vi "KelvinoxMonitor.vi"() -> ()   [LabVIEW 2019]
uses:
  Utility/Monitor Communication/Kelvinox/Kelvinox_Status_DD.ctl
  Global/Global Variables/Data_Display_global.vi
  Instrument_Setup.vi
panel:
  out "Kelvinox-Cluster":T1 {"Sorb Heater" format="%#.0f"; "Still Heater" format="%#.0f"; "MC Heater" format="%#.0f"; "T-Setpoint" format="%.3g"; "Sample" format="%_6g"; "4K" format="%_3g"; "MC" format="%_6g"; "Cold\nPlate" format="%_3g"; "1K Pot" format="%_3g"; "Still" format="%_3g"; "P5" format="%_3f"; "P4" format="%_3f"; "P3" format="%_3f"; "P2" format="%_3f"; "P1" format="%_3g"; "Dump" scale=0.0..1000.0}
  # "Hz"
  # "Temperatures in K"
  # "Resistances in Ohm"
  # "Pressures in mbar"
  # "Powers in µW"
  # "DU"
  # "He\nTrap"
  # "LN2\nTrap"
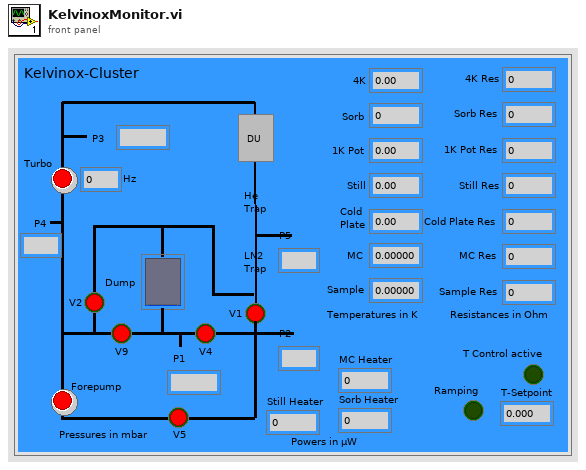
[diagram p1: front panel]
types:
  T1 = typedef "Kelvinox_Status_DD.ctl" = cluster{"V1":bool, "V2":bool, "Dump":u16, "V4":bool, "V5":bool, "V9":bool, "P1":dbl, "P2":dbl, "P3":dbl, "P4":dbl, "P5":dbl, "Turbo":bool, "Forepump":bool, "speed":dbl, "Sorb":dbl, "1K Pot":dbl, "Still":dbl, "Cold\nPlate":dbl, "MC":dbl, "4K":dbl, "Sample":dbl, "T-Setpoint":dbl, "MC Heater":dbl, "Still Heater":dbl, "Sorb Heater":dbl, "T Control active":bool, "Sorb Res":dbl, "1K Pot Res":dbl, "Still Res":dbl, "Cold Plate Res":dbl, "MC Res":dbl, "4K Res":dbl, "Sample Res":dbl, "Ramping":bool}
  T2 = cluster{"Mode":enum16{"Standard", "Buffered", "CRLF", "Immediate"}, "Bytes to Read":i32, "IP Address":string, "Remote Port":u16, "Timeout":i32, "connection ID":refnum<k5>}
  T3 = typedef "Kelvinox_Status.ctl" = cluster{"V1":bool, "V2":bool, "Dump":u16, "V4":bool, "V5":bool, "V9":bool, "P1":dbl, "P2":dbl, "P3":dbl, "P4":dbl, "P5":dbl, "Turbo":bool, "Forepump":bool, "speed":dbl, "Sorb":dbl, "1K Pot":dbl, "Still":dbl, "Cold\nPlate":dbl, "MC":dbl, "4K":dbl, "Sample":dbl, "T-Setpoint":dbl, "MC Heater":dbl, "Still Heater":dbl, "Sorb Heater":dbl, "T Control active":bool, "Sorb Res":dbl, "1K Pot Res":dbl, "Still Res":dbl, "Cold Plate Res":dbl, "MC Res":dbl, "4K Res":dbl, "Sample Res":dbl, "Ramping":bool}
  T4 = cluster{"Mode":enum16{"Standard", "Buffered", "CRLF", "Immediate"}, "Bytes to Read":i32, "IP Address":string, "Remote Port":i32, "Timeout":i32, "connection ID":refnum<k5>}
  T5 = typedef "Kelvinox_Control.ctl" = cluster{"T-Setpoint-Manual":dbl, "Rate (K/min)":dbl, "Change T Control Status":bool, "Emergency Stop":bool, "Set Setpoint":bool}
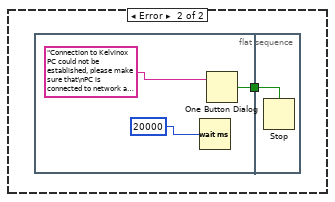
[diagram p2: hidden frame]
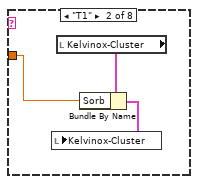
[diagram p4: hidden frame]
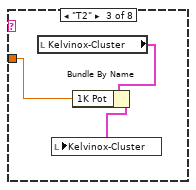
[diagram p5: hidden frame]
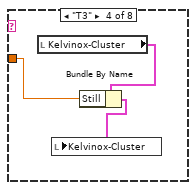
[diagram p6: hidden frame]
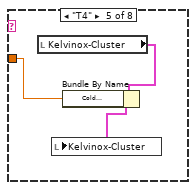
[diagram p7: hidden frame]
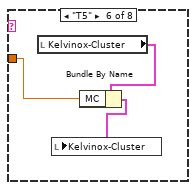
[diagram p8: hidden frame]
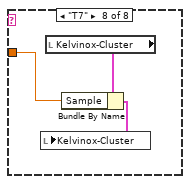
[diagram p9: hidden frame]
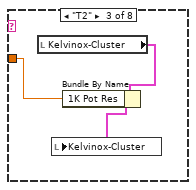
[diagram p11: hidden frame]
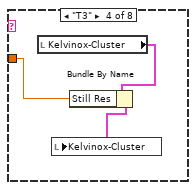
[diagram p12: hidden frame]
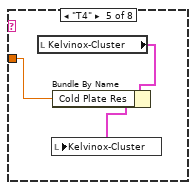
[diagram p13: hidden frame]
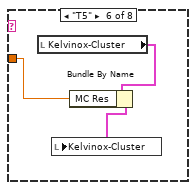
[diagram p14: hidden frame]
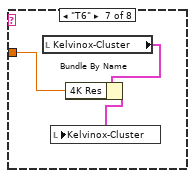
[diagram p15: hidden frame]
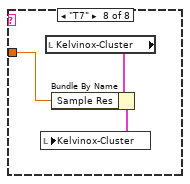
[diagram p16: hidden frame]
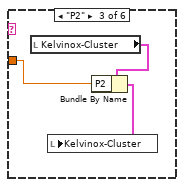
[diagram p18: hidden frame]
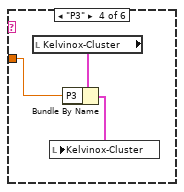
[diagram p19: hidden frame]
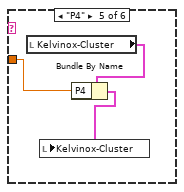
[diagram p20: hidden frame]
diagram:
  n1 = flat-sequence {
    tunnel: [w5] -> w3
    tunnel: [w4] -> w2
    tunnel: w3 -> [w14]
    tunnel: w2 -> [w13]
    tunnel: [w13] -> w1
    tunnel: w1 -> [w424]
    frame #0 {
      # "Establish TCP Connection"
      n2 = global read "Instrument_Setup.vi" "Connection Details Kelvinox"() -> (w6:T2)
      n3 = global read "Data_Display_global.vi" "Kelvinox-Cluster"() -> (→"Kelvinox-Cluster":T3)
      n4 = call "TRITON_RI_OPEN.vi"("Connection Details (in)"=w6) -> ("error out"=w5:errorcluster, "Connection Details (out)"=w4:T4)  [unwired: 2 in]
      n5 = case shown="No Error" w5 {
        frame No Error {
        }
        frame Error {
          n6 = flat-sequence {
            tunnel: [w9] -> w8
            tunnel: w8 -> [w12]
            frame #0 {
              n7 = Wait (ms)(milliseconds to wait=20000) -> ()  [unwired: 1 out]
              n8 = One Button Dialog(message="Connection to Kelvinox PC could not be established, please make sure that\nPC is connected to network and Triton control software is running.\n\nThe Kelvinox monitor will be restarted in 20 seconds if the status monitor is not stopped meanwhile.") -> (true=w9:bool)  [unwired: 1 in]
            }
            frame #1 {
              n9 = Stop(stop? (T)=w12) -> ()
            }
          }
        }
      }
    }
    frame #1 {
      n10 = while {
        tunnel: w14 -> [w40]
        tunnel: w13 -> [w41]
        stop <- w37 stop-if-true
        n11 = flat-sequence {
          tunnel: [w48] -> w36
          tunnel: [w50] -> w34
          tunnel: w40 -> [w49]
          tunnel: w41 -> [w50]
          tunnel: w36 -> [w89]
          tunnel: [w86] -> w35
          tunnel: w34 -> [w88]
          tunnel: [w88] -> w33
          tunnel: [w125] -> w47
          tunnel: [w124] -> w46
          tunnel: w35 -> [w126]
          tunnel: w33 -> [w124]
          tunnel: w47 -> [w161]
          tunnel: w46 -> [w158]
          tunnel: [w158] -> w45
          tunnel: [w157] -> w44
          tunnel: w45 -> [w195]
          tunnel: w44 -> [w199]
          tunnel: [w195] -> w43
          tunnel: [w193] -> w42
          tunnel: w43 -> [w206]
          tunnel: w42 -> [w210]
          tunnel: [w206] -> w32
          tunnel: [w205] -> w30
          tunnel: [w204] -> w28
          tunnel: w32 -> [w220]
          tunnel: [w220] -> w31
          tunnel: w30 -> [w216]
          tunnel: [w215] -> w29
          tunnel: w28 -> [w217]
          tunnel: w31 -> [w228]
          tunnel: [w228] -> w39
          tunnel: w29 -> [w230]
          tunnel: [w227] -> w38
          tunnel: w39 -> [w256]
          tunnel: [w256] -> w21
          tunnel: w38 -> [w257]
          tunnel: [w255] -> w19
          tunnel: [w254] -> w17
          tunnel: w21 -> [w266]
          tunnel: [w266] -> w20
          tunnel: w19 -> [w267]
          tunnel: [w268] -> w18
          tunnel: w17 -> [w269]
          tunnel: [w269] -> w16
          tunnel: [w264] -> w15
          tunnel: w20 -> [w282]
          tunnel: [w282] -> w25
          tunnel: w18 -> [w280]
          tunnel: [w281] -> w23
          tunnel: w16 -> [w283]
          tunnel: w15 -> [w276]
          tunnel: w25 -> [w292]
          tunnel: [w292] -> w24
          tunnel: w23 -> [w294]
          tunnel: [w293] -> w22
          tunnel: w24 -> [w388]
          tunnel: [w388] -> w27
          tunnel: w22 -> [w393]
          tunnel: [w395] -> w26
          tunnel: w27 -> [_]
          tunnel: w26 -> [w413]
          frame #0 {
            w51 = string[] ["T1", "T2", "T3", "T4", "T5", "T6", "T7"]
            # "Read Temperature Sensors"
            n12 = Array Size(array=w51) -> (size(s)=w52:i32)
            n13 = for {
              N: w52 -> [_]
              tunnel: w51 -> [w55] mode=indexing
              tunnel: w50 -> [w58]
              shift-right: [w56] -> w48
              shift-left: w49 -> [w57]
              n14 = Concatenate Strings("READ:DEV:", w55, ":TEMP:SIG:TEMP", "\r\n") -> (w64:string)
              n15 = call "TRITON_SEND_RECEIVE.vi"("error in (no error)"=w57, "Command String"=w64, "Communication Cluster"=w58) -> ("error out"=w60:errorcluster, "Response String"=w59:string)  [unwired: 1 in]
              n16 = call "TRITON_GET_VALUE.vi"("error in (no error)"=w60, "Response String"=w59) -> ("error out"=w56:errorcluster, "Value"=w54:dbl)  [unwired: 1 in, 1 out]
              n17 = case shown="\"T6\"" w55 {
                tunnel: w54 -> [_ w65 w68 w71 w74 w77 w82 w85]
                frame "empty", Default {
                }
                frame "T1" {
                  n18 = local read "Kelvinox-Cluster"() -> (w67:T1)
                  n19 = Bundle By Name(cluster=w67, "Sorb"=w65) -> (w66:T1)
                  n20 = local write "Kelvinox-Cluster"(w66) -> ()
                }
                frame "T2" {
                  n21 = local read "Kelvinox-Cluster"() -> (w70:T1)
                  n22 = Bundle By Name(cluster=w70, "1K Pot"=w68) -> (w69:T1)
                  n23 = local write "Kelvinox-Cluster"(w69) -> ()
                }
                frame "T3" {
                  n24 = local read "Kelvinox-Cluster"() -> (w73:T1)
                  n25 = Bundle By Name(cluster=w73, "Still"=w71) -> (w72:T1)
                  n26 = local write "Kelvinox-Cluster"(w72) -> ()
                }
                frame "T4" {
                  n27 = local read "Kelvinox-Cluster"() -> (w76:T1)
                  n28 = Bundle By Name(cluster=w76, "Cold\nPlate"=w74) -> (w75:T1)
                  n29 = local write "Kelvinox-Cluster"(w75) -> ()
                }
                frame "T5" {
                  n30 = local read "Kelvinox-Cluster"() -> (w79:T1)
                  n31 = Bundle By Name(cluster=w79, "MC"=w77) -> (w78:T1)
                  n32 = local write "Kelvinox-Cluster"(w78) -> ()
                }
                frame "T6" {
                  n33 = local read "Kelvinox-Cluster"() -> (w81:T1)
                  n34 = Bundle By Name(cluster=w81, "4K"=w82) -> (w80:T1)
                  n35 = local write "Kelvinox-Cluster"(w80) -> ()
                }
                frame "T7" {
                  n36 = local read "Kelvinox-Cluster"() -> (w84:T1)
                  n37 = Bundle By Name(cluster=w84, "Sample"=w85) -> (w83:T1)
                  n38 = local write "Kelvinox-Cluster"(w83) -> ()
                }
              }
              n39 = Wait (ms)(milliseconds to wait=10) -> ()  [unwired: 1 out]
            }
          }
          frame #1 {
            w87 = string[] ["T1", "T2", "T3", "T4", "T5", "T6", "T7"]
            # "Read Temperature Sensor Resistances"
            n40 = Array Size(array=w87) -> (size(s)=w90:i32)
            n41 = for {
              N: w90 -> [_]
              tunnel: w87 -> [w93] mode=indexing
              tunnel: w88 -> [w96]
              shift-right: [w94] -> w86
              shift-left: w89 -> [w95]
              n42 = Concatenate Strings("READ:DEV:", w93, ":TEMP:SIG:RES", "\r\n") -> (w102:string)
              n43 = call "TRITON_SEND_RECEIVE.vi"("error in (no error)"=w95, "Command String"=w102, "Communication Cluster"=w96) -> ("error out"=w98:errorcluster, "Response String"=w97:string)  [unwired: 1 in]
              n44 = call "TRITON_GET_VALUE.vi"("error in (no error)"=w98, "Response String"=w97) -> ("error out"=w94:errorcluster, "Value"=w92:dbl)  [unwired: 1 in, 1 out]
              n45 = case shown="\"T1\"" w93 {
                tunnel: w92 -> [_ w103 w106 w109 w112 w115 w120 w123]
                frame "empty", Default {
                }
                frame "T1" {
                  n46 = local read "Kelvinox-Cluster"() -> (w105:T1)
                  n47 = Bundle By Name(cluster=w105, "Sorb Res"=w103) -> (w104:T1)
                  n48 = local write "Kelvinox-Cluster"(w104) -> ()
                }
                frame "T2" {
                  n49 = local read "Kelvinox-Cluster"() -> (w108:T1)
                  n50 = Bundle By Name(cluster=w108, "1K Pot Res"=w106) -> (w107:T1)
                  n51 = local write "Kelvinox-Cluster"(w107) -> ()
                }
                frame "T3" {
                  n52 = local read "Kelvinox-Cluster"() -> (w111:T1)
                  n53 = Bundle By Name(cluster=w111, "Still Res"=w109) -> (w110:T1)
                  n54 = local write "Kelvinox-Cluster"(w110) -> ()
                }
                frame "T4" {
                  n55 = local read "Kelvinox-Cluster"() -> (w114:T1)
                  n56 = Bundle By Name(cluster=w114, "Cold Plate Res"=w112) -> (w113:T1)
                  n57 = local write "Kelvinox-Cluster"(w113) -> ()
                }
                frame "T5" {
                  n58 = local read "Kelvinox-Cluster"() -> (w117:T1)
                  n59 = Bundle By Name(cluster=w117, "MC Res"=w115) -> (w116:T1)
                  n60 = local write "Kelvinox-Cluster"(w116) -> ()
                }
                frame "T6" {
                  n61 = local read "Kelvinox-Cluster"() -> (w119:T1)
                  n62 = Bundle By Name(cluster=w119, "4K Res"=w120) -> (w118:T1)
                  n63 = local write "Kelvinox-Cluster"(w118) -> ()
                }
                frame "T7" {
                  n64 = local read "Kelvinox-Cluster"() -> (w122:T1)
                  n65 = Bundle By Name(cluster=w122, "Sample Res"=w123) -> (w121:T1)
                  n66 = local write "Kelvinox-Cluster"(w121) -> ()
                }
              }
              n67 = Wait (ms)(milliseconds to wait=10) -> ()  [unwired: 1 out]
            }
          }
          frame #2 {
            w128 = string[] ["P1", "P2", "P3", "P4", "P5"]
            # "Read Pressure Sensors"
            n68 = Array Size(array=w128) -> (size(s)=w127:i32)
            n69 = for {
              N: w127 -> [_]
              tunnel: w128 -> [w135] mode=indexing
              tunnel: w124 -> [w137]
              shift-right: [w132] -> w125
              shift-left: w126 -> [w136]
              n70 = Concatenate Strings("READ:DEV:", w135, ":PRES:SIG:PRES", "\r\n") -> (w140:string)
              n71 = call "TRITON_SEND_RECEIVE.vi"("error in (no error)"=w136, "Command String"=w140, "Communication Cluster"=w137) -> ("error out"=w133:errorcluster, "Response String"=w130:string)  [unwired: 1 in]
              n72 = call "TRITON_GET_VALUE.vi"("error in (no error)"=w133, "Response String"=w130) -> ("error out"=w132:errorcluster, "Value"=w131:dbl)  [unwired: 1 in, 1 out]
              n73 = case shown="\"P1\"" w135 {
                tunnel: w131 -> [_ w142 w145 w149 w151 w154]
                frame "empty", Default {
                }
                frame "P1" {
                  # "Nominal Dump\npressure:\n0.755 bar"
                  n74 = local read "Kelvinox-Cluster"() -> (w144:T1)
                  n75 = To Unsigned Word Integer(number=w142) -> (unsigned 16bit integer=w141:u16)
                  n76 = Bundle By Name(cluster=w144, "P1"=w142, "Dump"=w141) -> (w143:T1)
                  n77 = local write "Kelvinox-Cluster"(w143) -> ()
                }
                frame "P2" {
                  n78 = local read "Kelvinox-Cluster"() -> (w147:T1)
                  n79 = Bundle By Name(cluster=w147, "P2"=w145) -> (w146:T1)
                  n80 = local write "Kelvinox-Cluster"(w146) -> ()
                }
                frame "P3" {
                  n81 = local read "Kelvinox-Cluster"() -> (w150:T1)
                  n82 = Bundle By Name(cluster=w150, "P3"=w149) -> (w148:T1)
                  n83 = local write "Kelvinox-Cluster"(w148) -> ()
                }
                frame "P4" {
                  n84 = local read "Kelvinox-Cluster"() -> (w153:T1)
                  n85 = Bundle By Name(cluster=w153, "P4"=w151) -> (w152:T1)
                  n86 = local write "Kelvinox-Cluster"(w152) -> ()
                }
                frame "P5" {
                  n87 = local read "Kelvinox-Cluster"() -> (w156:T1)
                  n88 = Bundle By Name(cluster=w156, "P5"=w154) -> (w155:T1)
                  n89 = local write "Kelvinox-Cluster"(w155) -> ()
                }
              }
              n90 = Wait (ms)(milliseconds to wait=10) -> ()  [unwired: 1 out]
            }
          }
          frame #3 {
            w160 = string[] ["V1", "V2", "V4", "V5", "V9"]
            # "Read Valve States"
            n91 = Array Size(array=w160) -> (size(s)=w159:i32)
            n92 = for {
              N: w159 -> [_]
              shift-right: [w164] -> w157
              shift-left: w161 -> [w170]
              tunnel: w160 -> [w168] mode=indexing
              tunnel: w158 -> [w171]
              n93 = Concatenate Strings("READ:DEV:", w168, ":VALV:SIG:STATE", "\r\n") -> (w174:string)
              n94 = call "TRITON_SEND_RECEIVE.vi"("error in (no error)"=w170, "Command String"=w174, "Communication Cluster"=w171) -> ("error out"=w165:errorcluster, "Response String"=w166:string)  [unwired: 1 in]
              n95 = call "TRITON_GET_STATUS.vi"("error in (no error)"=w165, "Response String"=w166) -> ("error out"=w164:errorcluster, "Status"=w163:string)  [unwired: 2 in]
              n96 = call "Parse_Valve.vi"("Valve"=w163) -> ("Status"=w167:bool)
              n97 = case shown="\"V1\"" w168 {
                tunnel: w167 -> [w175 w178 w181 w184 w187 _]
                frame "V1" {
                  n98 = local read "Kelvinox-Cluster"() -> (w177:T1)
                  n99 = Bundle By Name(cluster=w177, "V1"=w175) -> (w176:T1)
                  n100 = local write "Kelvinox-Cluster"(w176) -> ()
                }
                frame "V2" {
                  n101 = local read "Kelvinox-Cluster"() -> (w180:T1)
                  n102 = Bundle By Name(cluster=w180, "V2"=w178) -> (w179:T1)
                  n103 = local write "Kelvinox-Cluster"(w179) -> ()
                }
                frame "V4" {
                  n104 = local read "Kelvinox-Cluster"() -> (w183:T1)
                  n105 = Bundle By Name(cluster=w183, "V4"=w181) -> (w182:T1)
                  n106 = local write "Kelvinox-Cluster"(w182) -> ()
                }
                frame "V5" {
                  n107 = local read "Kelvinox-Cluster"() -> (w186:T1)
                  n108 = Bundle By Name(cluster=w186, "V5"=w184) -> (w185:T1)
                  n109 = local write "Kelvinox-Cluster"(w185) -> ()
                }
                frame "V9" {
                  n110 = local read "Kelvinox-Cluster"() -> (w189:T1)
                  n111 = Bundle By Name(cluster=w189, "V9"=w187) -> (w188:T1)
                  n112 = local write "Kelvinox-Cluster"(w188) -> ()
                }
                frame "empty", Default {
                }
              }
              n113 = Wait (ms)(milliseconds to wait=10) -> ()  [unwired: 1 out]
            }
          }
          frame #4 {
            # "Read Forepump Status"
            n114 = Concatenate Strings("READ:DEV:FP:PUMP:SIG:STATE", "\r\n") -> (w202:string)
            n115 = call "TRITON_SEND_RECEIVE.vi"("error in (no error)"=w199, "Command String"=w202, "Communication Cluster"=w195) -> ("error out"=w194:errorcluster, "Response String"=w192:string)  [unwired: 1 in]
            n116 = call "TRITON_GET_STATUS.vi"("error in (no error)"=w194, "Response String"=w192) -> ("error out"=w193:errorcluster, "Status"=w191:string)  [unwired: 2 in]
            n117 = call "Parse_Valve.vi"("Valve"=w191) -> ("Status"=w197:bool)
            n118 = local read "Kelvinox-Cluster"() -> (w198:T1)
            n119 = Bundle By Name(cluster=w198, "Forepump"=w197) -> (w196:T1)
            n120 = local write "Kelvinox-Cluster"(w196) -> ()
            n121 = Wait (ms)(milliseconds to wait=10) -> ()  [unwired: 1 out]
          }
          frame #5 {
            # "Read Turbo Status"
            n122 = Concatenate Strings("READ:DEV:TURB1:PUMP:SIG:STATE", "\r\n") -> (w213:string)
            n123 = call "TRITON_SEND_RECEIVE.vi"("error in (no error)"=w210, "Command String"=w213, "Communication Cluster"=w206) -> ("error out"=w208:errorcluster, "Response String"=w209:string)  [unwired: 1 in]
            n124 = call "TRITON_GET_STATUS.vi"("error in (no error)"=w208, "Response String"=w209) -> ("error out"=w205:errorcluster, "Status"=w207:string)  [unwired: 2 in]
            n125 = call "Parse_Valve.vi"("Valve"=w207) -> ("Status"=w204:bool)
            n126 = Wait (ms)(milliseconds to wait=10) -> ()  [unwired: 1 out]
          }
          frame #6 {
            # "Read Turbo Speed"
            n127 = Concatenate Strings("READ:DEV:TURB1:PUMP:SIG:SPD", "\r\n") -> (w221:string)
            n128 = call "TRITON_SEND_RECEIVE.vi"("error in (no error)"=w216, "Command String"=w221, "Communication Cluster"=w220) -> ("error out"=w222:errorcluster, "Response String"=w223:string)  [unwired: 1 in]
            n129 = local read "Kelvinox-Cluster"() -> (w219:T1)
            n130 = call "TRITON_GET_VALUE.vi"("error in (no error)"=w222, "Response String"=w223) -> ("error out"=w215:errorcluster, "Value"=w224:dbl)  [unwired: 1 in, 1 out]
            n131 = Bundle By Name(cluster=w219, "Turbo"=w217, "speed"=w224) -> (w218:T1)
            n132 = local write "Kelvinox-Cluster"(w218) -> ()
            n133 = Wait (ms)(milliseconds to wait=10) -> ()  [unwired: 1 out]
          }
          frame #7 {
            w229 = string[] ["H1", "H2", "H3"]
            # "Read Heater Outputs"
            n134 = Array Size(array=w229) -> (size(s)=w231:i32)
            n135 = for {
              N: w231 -> [_]
              shift-right: [w237] -> w227
              shift-left: w230 -> [w239]
              tunnel: w229 -> [w234] mode=indexing
              tunnel: w228 -> [w238]
              n136 = Concatenate Strings("READ:DEV:", w234, ":HTR:SIG:POWR", "\r\n") -> (w243:string)
              n137 = call "TRITON_SEND_RECEIVE.vi"("error in (no error)"=w239, "Command String"=w243, "Communication Cluster"=w238) -> ("error out"=w236:errorcluster, "Response String"=w235:string)  [unwired: 1 in]
              n138 = call "TRITON_GET_VALUE.vi"("error in (no error)"=w236, "Response String"=w235) -> ("error out"=w237:errorcluster, "Value"=w233:dbl)  [unwired: 1 in, 1 out]
              n139 = case shown="\"H3\"" w234 {
                tunnel: w233 -> [w244 w247 w251 _]
                frame "H1" {
                  n140 = local read "Kelvinox-Cluster"() -> (w246:T1)
                  n141 = Bundle By Name(cluster=w246, "MC Heater"=w244) -> (w245:T1)
                  n142 = local write "Kelvinox-Cluster"(w245) -> ()
                }
                frame "H2" {
                  n143 = local read "Kelvinox-Cluster"() -> (w249:T1)
                  n144 = Bundle By Name(cluster=w249, "Still Heater"=w247) -> (w248:T1)
                  n145 = local write "Kelvinox-Cluster"(w248) -> ()
                }
                frame "H3" {
                  n146 = local read "Kelvinox-Cluster"() -> (w252:T1)
                  n147 = Bundle By Name(cluster=w252, "Sorb Heater"=w251) -> (w250:T1)
                  n148 = local write "Kelvinox-Cluster"(w250) -> ()
                }
                frame "empty", Default {
                }
              }
              n149 = Wait (ms)(milliseconds to wait=10) -> ()  [unwired: 1 out]
            }
          }
          frame #8 {
            # "Read Temperature Control"
            n150 = Concatenate Strings("READ:DEV:T5:TEMP:LOOP:MODE", "\r\n") -> (w263:string)
            n151 = call "TRITON_SEND_RECEIVE.vi"("error in (no error)"=w257, "Command String"=w263, "Communication Cluster"=w256) -> ("error out"=w259:errorcluster, "Response String"=w260:string)  [unwired: 1 in]
            n152 = call "TRITON_GET_STATUS.vi"("error in (no error)"=w259, "Response String"=w260) -> ("error out"=w255:errorcluster, "Status"=w258:string)  [unwired: 2 in]
            n153 = call "Parse_Valve.vi"("Valve"=w258) -> ("Status"=w254:bool)
            n154 = Wait (ms)(milliseconds to wait=10) -> ()  [unwired: 1 out]
          }
          frame #9 {
            # "Read Ramping Status"
            n155 = Concatenate Strings("READ:DEV:T5:TEMP:LOOP:RAMP:RAMPING", "\r\n") -> (w275:string)
            n156 = call "TRITON_SEND_RECEIVE.vi"("error in (no error)"=w267, "Command String"=w275, "Communication Cluster"=w266) -> ("error out"=w271:errorcluster, "Response String"=w272:string)  [unwired: 1 in]
            n157 = call "TRITON_GET_STATUS.vi"("error in (no error)"=w271, "Response String"=w272) -> ("error out"=w268:errorcluster, "Status"=w265:string)  [unwired: 2 in]
            n158 = Wait (ms)(milliseconds to wait=10) -> ()  [unwired: 1 out]
            n159 = call "Parse_Valve.vi"("Valve"=w265) -> ("Status"=w264:bool)
          }
          frame #10 {
            # "Read Temperature Control Setpoint"
            n160 = Concatenate Strings("READ:DEV:T5:TEMP:LOOP:TSET", "\r\n") -> (w289:string)
            n161 = call "TRITON_SEND_RECEIVE.vi"("error in (no error)"=w280, "Command String"=w289, "Communication Cluster"=w282) -> ("error out"=w284:errorcluster, "Response String"=w285:string)  [unwired: 1 in]
            n162 = local read "Kelvinox-Cluster"() -> (w279:T1)
            n163 = call "TRITON_GET_VALUE.vi"("error in (no error)"=w284, "Response String"=w285) -> ("error out"=w281:errorcluster, "Value"=w286:dbl)  [unwired: 1 in, 1 out]
            n164 = Bundle By Name(cluster=w279, "T Control active"=w283, "Ramping"=w276, "T-Setpoint"=w286) -> (w278:T1)
            n165 = local write "Kelvinox-Cluster"(w278) -> ()
            n166 = Wait (ms)(milliseconds to wait=10) -> ()  [unwired: 1 out]
          }
          frame #11 {
            # "ToDo: Implement Thermometer excitation and range"
            # "Change Heater Range if Loop mode is enabled"
            n167 = local read "Kelvinox-Cluster"() -> (w295:T1)
            n168 = Unbundle By Name(w295) -> ("T-Setpoint"=w290:dbl, "T Control active"=w291:bool)
            n169 = case shown="True" w291 {
              tunnel: w294 -> [w296 w311]
              tunnel: [w296 w310] -> w293
              tunnel: w292 -> [_ w309]
              tunnel: w290 -> [_ w306]
              frame False {
              }
              frame True {
                n170 = stacked-sequence {
                  seq-local: [w314 _ _ _] -> [_ w324 _ _]
                  seq-local: [_ w323 _ _] -> [_ _ w331 _]
                  seq-local: [_ _ w330 _] -> [_ _ _ w339]
                  tunnel: w311 -> [w319 _ _ _]
                  tunnel: w309 -> [w315 w322 w329 w337]
                  tunnel: [_ w320 _ _] -> w303
                  tunnel: [w312 _ _ _] -> w304
                  tunnel: [_ _ w328 _] -> w302
                  tunnel: [_ _ _ w336] -> w307
                  tunnel: [_ _ _ w338] -> w301
                  frame #0 {
                    n171 = Concatenate Strings("READ:DEV:T5:TEMP:LOOP:RANGE", "\r\n") -> (w316:string)
                    n172 = call "TRITON_SEND_RECEIVE.vi"("error in (no error)"=w319, "Command String"=w316, "Communication Cluster"=w315) -> ("error out"=w314:errorcluster, "Response String"=w313:string)  [unwired: 1 in]
                    n173 = call "Kelvinox_Parse_Heater_Excitation_to_Number.vi"("Excitation String"=w313) -> ("Excitation Level"=w312:dbl)
                  }
                  frame #1 {
                    n174 = Concatenate Strings("READ:DEV:T5:TEMP:LOOP:P", "\r\n") -> (w325:string)
                    n175 = call "TRITON_SEND_RECEIVE.vi"("error in (no error)"=w324, "Command String"=w325, "Communication Cluster"=w322) -> ("error out"=w323:errorcluster, "Response String"=w321:string)  [unwired: 1 in]
                    n176 = call "Kelvinox_Parse_PID_to_Number.vi"("PID String"=w321) -> ("PID Number"=w320:dbl)
                  }
                  frame #2 {
                    n177 = Concatenate Strings("READ:DEV:T5:TEMP:LOOP:I", "\r\n") -> (w333:string)
                    n178 = call "TRITON_SEND_RECEIVE.vi"("error in (no error)"=w331, "Command String"=w333, "Communication Cluster"=w329) -> ("error out"=w330:errorcluster, "Response String"=w332:string)  [unwired: 1 in]
                    n179 = call "Kelvinox_Parse_PID_to_Number.vi"("PID String"=w332) -> ("PID Number"=w328:dbl)
                  }
                  frame #3 {
                    n180 = Concatenate Strings("READ:DEV:T5:TEMP:LOOP:D", "\r\n") -> (w341:string)
                    n181 = call "TRITON_SEND_RECEIVE.vi"("error in (no error)"=w339, "Command String"=w341, "Communication Cluster"=w337) -> ("error out"=w336:errorcluster, "Response String"=w340:string)  [unwired: 1 in]
                    n182 = call "Kelvinox_Parse_PID_to_Number.vi"("PID String"=w340) -> ("PID Number"=w338:dbl)
                  }
                }
                n183 = call "Kelvinox_set_zone_properties.vi"("Heater_range_old"=w304, "P_old"=w303, "I_old"=w302, "D_old"=w301, "Temperature Setpoint"=w306) -> ("Change?"=w305:bool, "Heater_range_new"=w300:dbl, "P_new"=w299:dbl, "I_new"=w298:dbl, "D_new"=w297:dbl)  [unwired: 10 in]
                n184 = case shown="True" w305 {
                  tunnel: w300 -> [_ w350]
                  tunnel: w307 -> [w344 w346]
                  tunnel: [w344 w345] -> w310
                  tunnel: w309 -> [_ w351]
                  tunnel: w299 -> [_ w349]
                  tunnel: w298 -> [_ w348]
                  tunnel: w297 -> [_ w347]
                  frame False {
                  }
                  frame True {
                    n185 = stacked-sequence {
                      seq-local: [w355 _ _ _] -> [_ w364 _ _]
                      seq-local: [_ w363 _ _] -> [_ _ w373 _]
                      seq-local: [_ _ w372 _] -> [_ _ _ w382]
                      tunnel: w351 -> [w358 w365 w374 w383]
                      tunnel: w350 -> [w353 _ _ _]
                      tunnel: w349 -> [_ w362 _ _]
                      tunnel: w348 -> [_ _ w371 _]
                      tunnel: w347 -> [_ _ _ w381]
                      tunnel: w346 -> [w354 _ _ _]
                      tunnel: [_ _ _ w379] -> w345
                      frame #0 {
                        n186 = call "Kelvinox_Parse_Heater_Number_to_Excitation.vi"("Excitation Level"=w353) -> ("Excitation String"=w352:string)
                        n187 = Concatenate Strings("SET:DEV:T5:TEMP:LOOP:RANGE", ":", w352, "\r\n") -> (w359:string)
                        n188 = call "TRITON_SEND_RECEIVE.vi"("error in (no error)"=w354, "Command String"=w359, "Communication Cluster"=w358) -> ("error out"=w355:errorcluster)  [unwired: 1 in, 1 out]
                      }
                      frame #1 {
                        n189 = Number To Engineering String(4:w362) -> (0:w361:string)  [unwired: 3 in]
                        n190 = Concatenate Strings("SET:DEV:T5:TEMP:LOOP:P", ":", w361, "\r\n") -> (w368:string)
                        n191 = call "TRITON_SEND_RECEIVE.vi"("error in (no error)"=w364, "Command String"=w368, "Communication Cluster"=w365) -> ("error out"=w363:errorcluster)  [unwired: 1 in, 1 out]
                      }
                      frame #2 {
                        n192 = Number To Engineering String(4:w371) -> (0:w370:string)  [unwired: 3 in]
                        n193 = Concatenate Strings("SET:DEV:T5:TEMP:LOOP:I", ":", w370, "\r\n") -> (w377:string)
                        n194 = call "TRITON_SEND_RECEIVE.vi"("error in (no error)"=w373, "Command String"=w377, "Communication Cluster"=w374) -> ("error out"=w372:errorcluster)  [unwired: 1 in, 1 out]
                      }
                      frame #3 {
                        n195 = Number To Engineering String(4:w381) -> (0:w380:string)  [unwired: 3 in]
                        n196 = Concatenate Strings("SET:DEV:T5:TEMP:LOOP:D", ":", w380, "\r\n") -> (w386:string)
                        n197 = call "TRITON_SEND_RECEIVE.vi"("error in (no error)"=w382, "Command String"=w386, "Communication Cluster"=w383) -> ("error out"=w379:errorcluster)  [unwired: 1 in, 1 out]
                      }
                    }
                  }
                }
                n198 = Wait (ms)(milliseconds to wait=10) -> ()  [unwired: 1 out]
              }
            }
          }
          frame #12 {
            # "TODO:\nFix readout error\nafter change loop\nmode"
            # "Write Values"
            n199 = call "Kelvinox_Open_Queue.vi"("error in (no error)"=w393) -> ("error out"=w392:errorcluster, "queue out"=w394:refnum<queue>)  [unwired: 9 in]
            n200 = call "Kelvinox_Check_Queue.vi"("error in (no error)"=w392, "queue"=w394) -> ("error out"=w391:errorcluster, "Kelvinox-Control"=w389:T5, "New Entries?"=w390:bool)  [unwired: 6 in]
            n201 = case shown="True" w390 {
              tunnel: w391 -> [w396 w400]
              tunnel: [w396 w397] -> w395
              tunnel: w389 -> [_ w399]
              tunnel: w388 -> [_ w398]
              frame False {
              }
              frame True {
                n202 = stacked-sequence {
                  seq-local: [w401 _] -> [_ w405]
                  tunnel: w400 -> [w404 _]
                  tunnel: w399 -> [w403 w409]
                  tunnel: w398 -> [w402 w408]
                  tunnel: [_ w407] -> w397
                  frame #0 {
                    n203 = call "Kelvinox_Set_T_Setpoint.vi"("error in (no error)"=w404, "Kelvinox-Cluster"=w403, "Connection Details (in)"=w402) -> ("error out"=w401:errorcluster)  [unwired: 8 in]
                  }
                  frame #1 {
                    n204 = call "Kelvinox_Change_Loop_Mode.vi"("error in (no error)"=w405, "Kelvinox-Cluster"=w409, "Connection Details (in)"=w408) -> ("error out"=w407:errorcluster)  [unwired: 8 in]
                    n205 = Wait (ms)(milliseconds to wait=10) -> ()  [unwired: 1 out]
                  }
                }
              }
            }
          }
          frame #13 {
            # "Write to Global Cluster"
            n206 = global read "Instrument_Setup.vi" "T-Sweep Control Thermometer"() -> (w412:u16)
            n207 = call "Error_handler.vi"("error constant"=w413) -> ()
            n208 = local read "Kelvinox-Cluster"() -> (w411:T1)
            n209 = case shown="1" w412 {
              tunnel: w411 -> [w414 w417]
              frame 0, Default {
                n210 = Unbundle By Name(w414) -> ("MC"=w416:dbl, "MC Res"=w415:dbl)
                n211 = global write "Data_Display_global.vi" "Control Temperature Resistance"(w415) -> ()
                n212 = global write "Data_Display_global.vi" "Control Temperature SC"(w416) -> ()
              }
              frame 1 {
                n213 = Unbundle By Name(w417) -> ("Sample"=w419:dbl, "Sample Res"=w418:dbl)
                n214 = global write "Data_Display_global.vi" "Control Temperature Resistance"(w418) -> ()
                n215 = global write "Data_Display_global.vi" "Control Temperature SC"(w419) -> ()
              }
            }
            n216 = Unbundle By Name(w411) -> ("Sample"=w410:dbl)
            n217 = global write "Data_Display_global.vi" "Sample Temperature 1 SC"(w410) -> ()
            n218 = global write "Data_Display_global.vi" "Kelvinox-Cluster"(w411) -> ()
          }
          frame #14 {
            # "Wait until readout time has passed"
            n219 = global read "Instrument_Setup.vi" "readout (s)"() -> (w422:dbl)
            n220 = Multiply(x=1000, y=w422) -> (x*y=w421:dbl)
            n221 = Wait (ms)(milliseconds to wait=w421) -> ()  [unwired: 1 out]
          }
        }
        n222 = global read "Data_Display_global.vi" "Stop Monitors"() -> (w37:bool)
      }
    }
    frame #2 {
      # "Close TCP connection"
      n223 = call "TRITON_RI_CLOSE.vi"("Communication Cluster"=w424) -> ("error out"=w423:errorcluster)  [unwired: 1 in]
      n224 = call "Error_handler.vi"("error constant"=w423) -> ()
    }
  }
